vi "personirijillas.vi"() -> ()   [LabVIEW 2013]
uses:
  <vilib>/silver_ctls/ArrayMatrixCluster/Real Matrix NI_Silver.ctl
panel:
  out "Real Matrix 2":T1
  out "Command":string
  out "5":bool
  out "4":bool
  out "3":bool
  out "2":bool
  out "1":bool
  out "Reconocida":dbl[](graph)
  out "Input Signal Energy":dbl
  out "Entrada":waveform(dbl)[](graph)
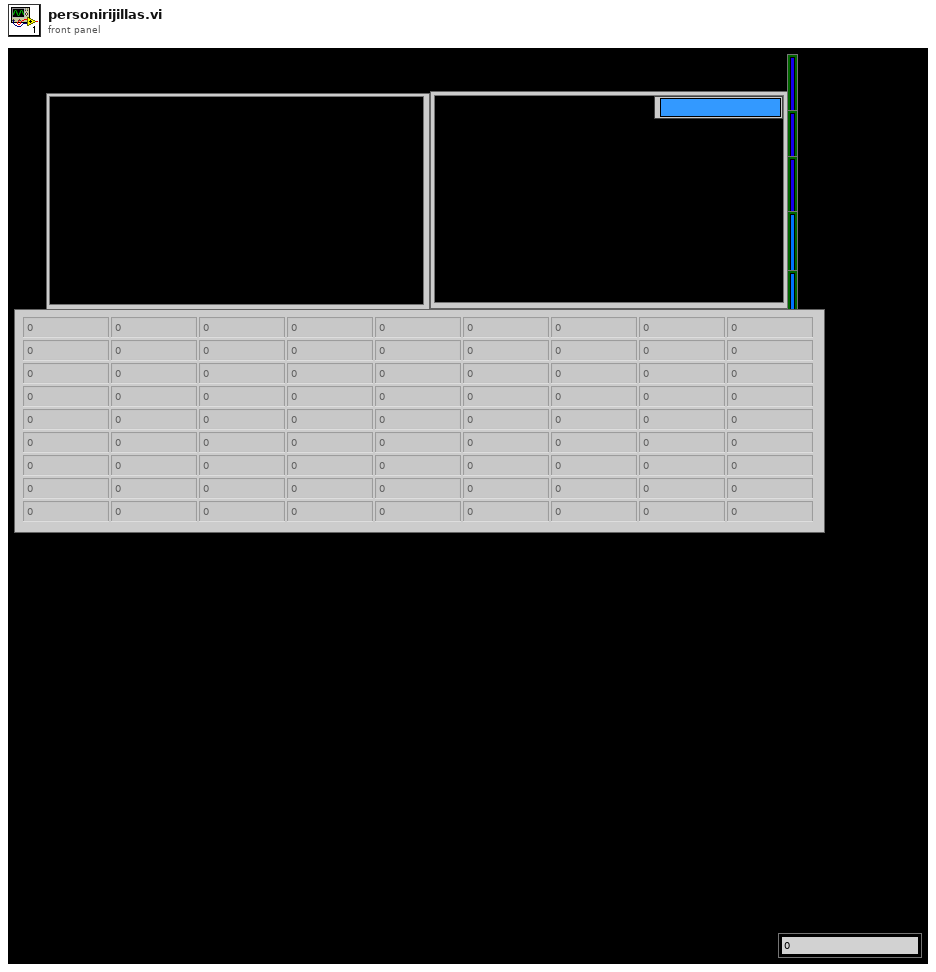
[diagram p1: front panel]
types:
  T1 = typedef "Real Matrix NI_Silver.ctl" = dbl[][]
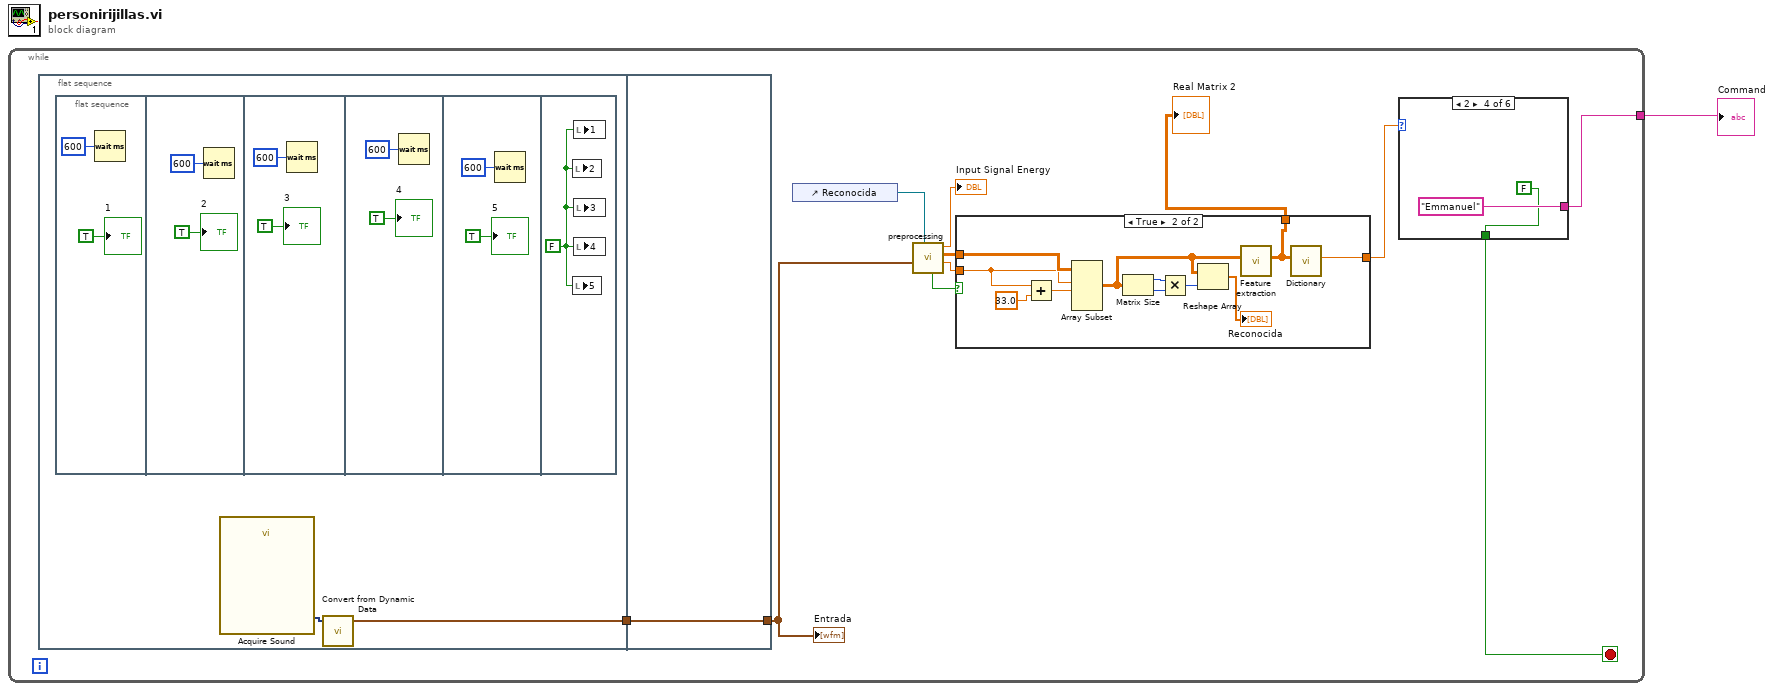
[diagram p0: block diagram]
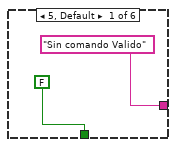
[diagram p2: hidden frame]
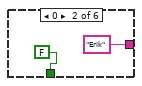
[diagram p3: hidden frame]
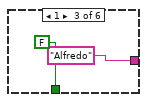
[diagram p4: hidden frame]
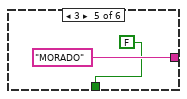
[diagram p5: hidden frame]
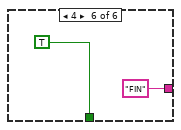
[diagram p6: hidden frame]
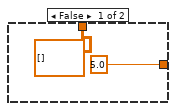
[diagram p7: hidden frame]
diagram:
  n1 = while {
    tunnel: [w2] -> w1
    stop <- w4 stop-if-true
    n2 = flat-sequence {
      tunnel: [w38] -> w8
      tunnel: [w51] -> w6
      tunnel: w8 -> [w51]
      frame #0 {
        n3 = flat-sequence {
          frame #0 {
            n4 = Wait (ms)(milliseconds to wait=u32 600) -> ()  [unwired: 1 out]
            "1" <- TRUE ("1")
          }
          frame #1 {
            n5 = Wait (ms)(milliseconds to wait=u32 600) -> ()  [unwired: 1 out]
            "2" <- TRUE ("1")
          }
          frame #2 {
            n6 = Wait (ms)(milliseconds to wait=u32 600) -> ()  [unwired: 1 out]
            "3" <- TRUE ("1")
          }
          frame #3 {
            n7 = Wait (ms)(milliseconds to wait=u32 600) -> ()  [unwired: 1 out]
            "4" <- TRUE ("1")
          }
          frame #4 {
            n8 = Wait (ms)(milliseconds to wait=u32 600) -> ()  [unwired: 1 out]
            "5" <- TRUE ("1")
          }
          frame #5 {
            w50 = FALSE ("1")
            n9 = local write "2"(w50) -> ()
            n10 = local write "5"(w50) -> ()
            n11 = local write "1"(w50) -> ()
            n12 = local write "3"(w50) -> ()
            n13 = local write "4"(w50) -> ()
          }
        }
        n14 = call "Acquire Sound"() -> ("Data"=w39:dynamicdata)  [unwired: 18 in, 1 out]
        n15 = call "Convert from Dynamic Data"("Dynamic Data Type"=w39) -> ("Array of Waveform"=w38:waveform(dbl)[])  [unwired: 3 in]
      }
      frame #1 {
      }
    }
    n16 = control-ref of="Reconocida"() -> (w5:refnum<vi>)
    n17 = call "preprocessing.vi"("WaveformGraph in"=w5, "Input Speech"=w6) -> ("Start index"=w11:dbl, "Frames"=w10:dbl[][], "Signal energy"=→"Input Signal Energy":dbl, "Boolean"=w12:bool)  [unwired: 6 in]
    n18 = case shown="True" w12 {
      tunnel: w11 -> [_ w30]
      tunnel: w10 -> [_ w31]
      tunnel: [5.0 ("Best Match") w29] -> w9
      tunnel: [dbl[][] [] ("Acoustic vector") w27] -> w3
      frame False {
      }
      frame True {
        n19 = Add(x=w30, y=33.0 ("x")) -> (x+y=w36:dbl)
        n20 = Array Subset(array=w31, index (row)=w30, length (row)=w36) -> (w28:dbl[][])  [unwired: 2 in]
        n21 = Matrix Size(0:w28) -> (1:w35:i32, 2:w34:i32)
        n22 = Multiply(x=w35, y=w34) -> (x*y=w33:i32)
        n23 = Reshape Array(w28, w33) -> (→"Reconocida":dbl[])
        n24 = call "Feature extraction.vi"("Utterance Frames"=w28) -> ("Acoustic vector"=w27:dbl[][])  [unwired: 10 in]
        n25 = call "Dictionary.vi"("Match Input"=w27) -> ("Best Match"=w29:dbl)  [unwired: 10 in]
      }
    }
    "Real Matrix 2" <- w3
    n26 = case shown="2" w9 {
      tunnel: ["Sin comando Valido" ("Command") "Erik" ("Command") "Alfredo" ("Command") "Emmanuel" ("Command") "MORADO" ("Command") "FIN" ("Command")] -> w2
      tunnel: [FALSE ("RIGHT") FALSE ("RIGHT") FALSE ("RIGHT") FALSE ("RIGHT") FALSE ("RIGHT") TRUE ("RIGHT")] -> w4
      frame 5, Default {
      }
      frame 0 {
      }
      frame 1 {
      }
      frame 2 {
      }
      frame 3 {
      }
      frame 4 {
      }
    }
    "Entrada" <- w6
  }
  "Command" <- w1
